vi "Get Array Combination Recursive.vi"(6 "Max Column Index":i32, 8 "Column":i32, 9 "Row":i32, 10 "Array":variant[](array[variant]), 11 "blankResultsIn":variant[][](array[variant])) -> (2 "Row Out":i32, 3 "Results Out":variant[][](array[variant]))   [LabVIEW 2016]
panel:
  # "#CrazyShit This VI calls itself!"
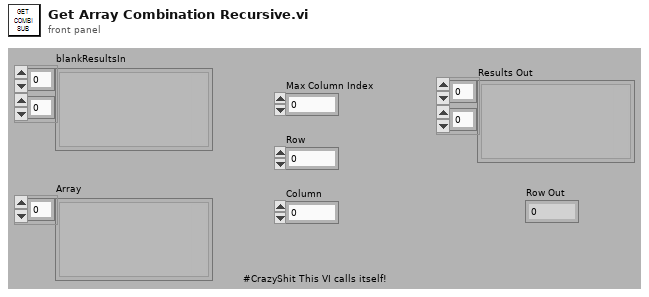
[diagram p1: front panel]
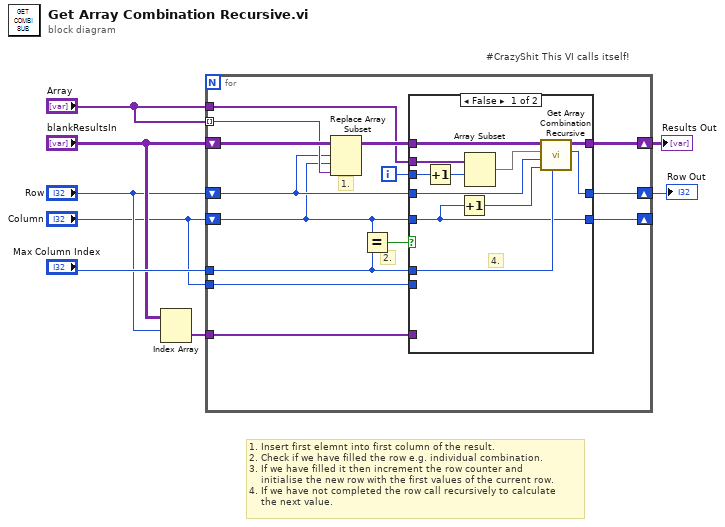
[diagram p0: block diagram]
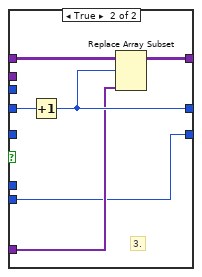
[diagram p2: hidden frame]
diagram:
  # "#CrazyShit This VI calls itself!"
  # "1. Insert first elemnt into first column of the result.\n2. Check if we have filled the row e.g. individual combination.\n3. If we have filled it then increment the row counter and \n    initialise the new row with the first values of the current row.\n4. If we have not completed the row call recursively to calculate\n    the next value."
  n1 = Index Array(array="blankResultsIn", index (row)="Row") -> (element=w2:variant[])  [unwired: 1 in]
  n2 = for {
    shift-right: [w15] -> w8
    shift-left: "blankResultsIn" -> [w22]
    tunnel: "Array" -> [w21] mode=indexing
    shift-right: [w18] -> w6
    shift-left: "Row" -> [w19]
    shift-right: [w17] -> _
    shift-left: "Column" -> [w14]
    tunnel: "Max Column Index" -> [w13]
    tunnel: "Array" -> [w12]
    tunnel: "Column" -> [w11]
    tunnel: w2 -> [w10]
    i -> [w9]
    # "2."
    # "1."
    n3 = Replace Array Subset(array=w22, new element=w21, index (row)=w19, index (col)=w14) -> (w16:variant[][])
    n4 = Equal?(x=w14, y=w13) -> (x = y?=w20:bool)
    n5 = case shown="False" w20 {
      tunnel: w19 -> [w26 w39]
      tunnel: [w31 w36] -> w18
      tunnel: [w23 w34] -> w17
      tunnel: w16 -> [w27 w38]
      tunnel: [w33 w37] -> w15
      tunnel: w14 -> [w23 _]
      tunnel: w13 -> [w32 _]
      tunnel: w12 -> [w30 _]
      tunnel: w11 -> [_ w34]
      tunnel: w10 -> [_ w35]
      tunnel: w9 -> [w24 _]
      frame False {
        # "4."
        n6 = Increment(x=w24) -> (x+1=w25:i32)
        n7 = Increment(x=w23) -> (x+1=w28:i32)
        n8 = Array Subset(array=w30, index=w25) -> (w29:variant[])  [unwired: 1 in]
        n9 = call "Get Array Combination Recursive.vi"("Max Column Index"=w32, "Column"=w28, "Row"=w26, "Array"=w29, "blankResultsIn"=w27) -> ("Row Out"=w31:i32, "Results Out"=w33:variant[][])  [unwired: 5 in]
      }
      frame True {
        # "3."
        n10 = Increment(x=w39) -> (x+1=w36:i32)
        n11 = Replace Array Subset(array=w38, new element=w35, index (row)=w36) -> (w37:variant[][])  [unwired: 1 in]
      }
    }
  }
  "Results Out" <- w8
  "Row Out" <- w6
